vi "rotation.vi"() -> (1 "appended array 3":T1, 2 "appended array 2":T1, 3 "appended array":T1)   [LabVIEW 2020]
uses:
  <vilib>/Analysis/Matrix/Datatypes/RealMatrix.ctl
  <vilib>/Analysis/Matrix/NI_Matrix.lvlib
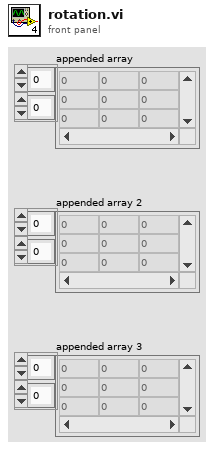
[diagram p1: front panel]
types:
  T1 = typedef "NI_Matrix.lvlib/RealMatrix.ctl" = dbl[][]
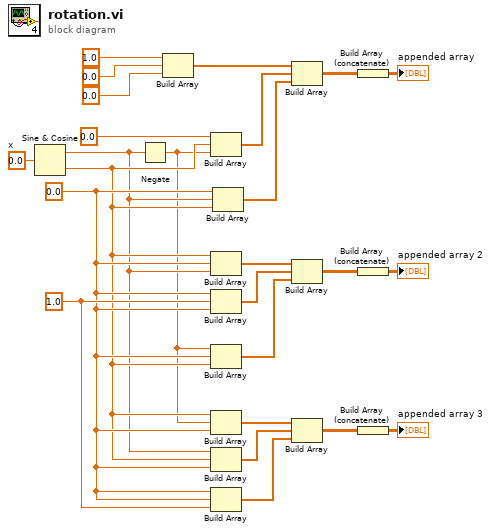
[diagram p0: block diagram]
diagram:
  w22 = 0.0  # x
  w17 = 1.0
  w16 = 0.0
  n1 = Sine & Cosine(0:w22) -> (1:w14:dbl, 2:w15:dbl)
  n2 = Negate(x=w14) -> (-x=w13:dbl)
  n3 = Build Array(1.0, 0.0, 0.0) -> (w5:dbl[])
  n4 = Build Array(0.0, w15, w13) -> (w6:dbl[])
  n5 = Build Array(w15, w16, w14) -> (w9:dbl[])
  n6 = Build Array(w16, w17, w16) -> (w10:dbl[])
  n7 = Build Array(w13, w16, w15) -> (w11:dbl[])
  n8 = Build Array(w15, w13, w16) -> (w18:dbl[])
  n9 = Build Array(w14, w15, w16) -> (w19:dbl[])
  n10 = Build Array(w16, w16, w17) -> (w20:dbl[])
  n11 = Build Array(w16, w14, w15) -> (w7:dbl[])
  n12 = Build Array(w5, w6, w7) -> (w8:dbl[][])
  n13 = Build Array(w9, w10, w11) -> (w12:dbl[][])
  n14 = Build Array(w18, w19, w20) -> (w21:dbl[][])
  n15 = Build Array (concatenate)(w8) -> (→"appended array":T1)
  n16 = Build Array (concatenate)(w12) -> (→"appended array 2":T1)
  n17 = Build Array (concatenate)(w21) -> (→"appended array 3":T1)
